vi "data save(1).vi"(8 "error in":errorcluster caption="Error In", 10 "保存时间间隔":u16(ring)=1 items=["无间隔"=1, "1分钟"=60, "5分钟"=300, "10分钟"=600, "30分钟"=1800, "1小时"=3600], 11 "CalData":T1(array[cluster])) -> (0 "error out":errorcluster caption="Error out")   [LabVIEW 2011]
panel:
  in  "targer":enum16{"主舱外回路", "主舱内回路", "实验舱外回路", "实验舱内回路"}(ring)
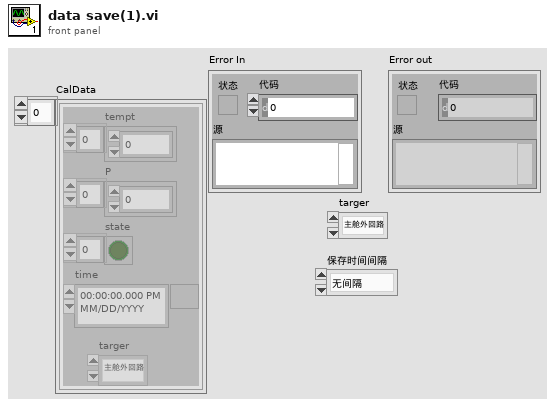
[diagram p1: front panel]
types:
  T1 = cluster{"tempt":dbl[], "P":dbl[], "state":bool[], "time":timestamp, "targer":enum16{"主舱外回路", "主舱内回路", "实验舱外回路", "实验舱内回路"}}[]
  T2 = typedef "Enum File IO - FGV(V)_Ctrls-某型振动实验台测试系统.ctl" = enum16{"New", "Open", "Write Info", "Write Data", "Read Info", "Read Chan Names", "Read Data", "Close", "None"}
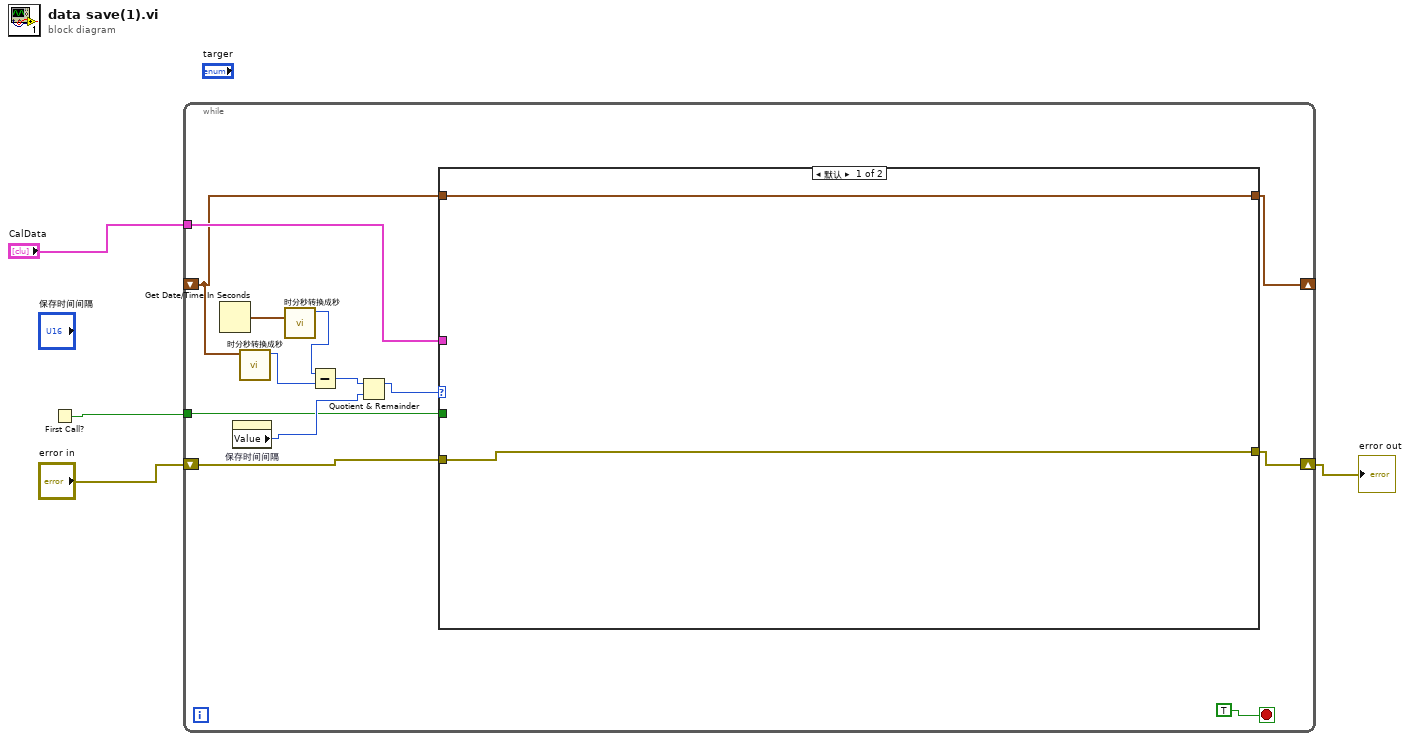
[diagram p0: block diagram]
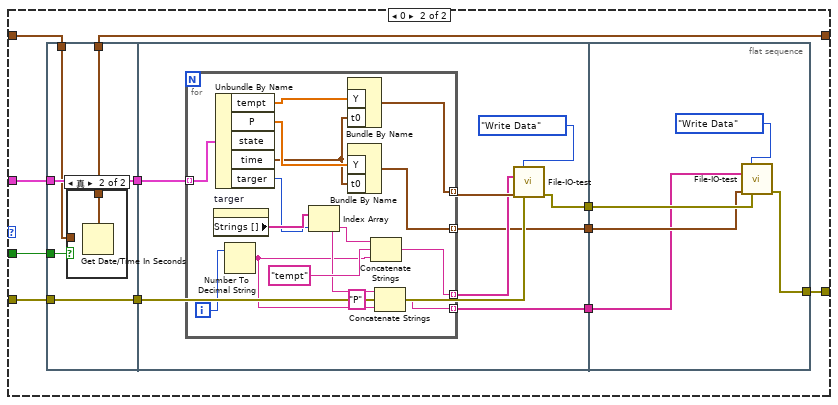
[diagram p2: hidden frame]
diagram:
  n1 = First Call?() -> (First Call?: T/F=w1:bool)
  n2 = while {
    tunnel: "CalData" -> [w17]
    shift-right: [w15] -> w2
    shift-left: "error in" -> [w16]
    shift-right: [w14] -> _
    shift-left: _ -> [w10]
    tunnel: w1 -> [w5]
    stop <- TRUE stop-if-true
    n3 = Get Date/Time In Seconds() -> (seconds since 1Jan1904=w12:timestamp)
    n4 = property on="保存时间间隔" class="Ring (严格)"() -> ("Value"=w7:u16)  [unwired: 2 in, 2 out]
    n5 = call "时分秒转换成秒.vi"("seconds since 1Jan1904"=w10) -> ("数值"=w9:i32)  [unwired: 10 in]
    n6 = call "时分秒转换成秒.vi"("seconds since 1Jan1904"=w12) -> ("数值"=w11:i32)  [unwired: 10 in]
    n7 = Subtract(x=w11, y=w9) -> (x-y=w8:i32)
    n8 = Quotient & Remainder(x=w8, y=w7) -> (x-y*floor(x/y)=w6:i32)  [unwired: 1 out]
    n9 = case shown="默认" w6 {
      tunnel: w17 -> [_ w27]
      tunnel: w16 -> [w19 w26]
      tunnel: [w19 w25] -> w15
      tunnel: [w18 w22] -> w14
      tunnel: w10 -> [w18 w20]
      tunnel: w5 -> [_ w21]
      frame Default {
      }
      frame 0 {
        n10 = flat-sequence {
          tunnel: w26 -> [w34]
          tunnel: w27 -> [w35]
          tunnel: [w35] -> w24
          tunnel: [w34] -> w23
          tunnel: [w32] -> w22
          tunnel: w21 -> [w33]
          tunnel: w20 -> [w31]
          tunnel: [w41] -> w30
          tunnel: [w39] -> w29
          tunnel: [w38] -> w28
          tunnel: w24 -> [w45]
          tunnel: w23 -> [w42]
          tunnel: w30 -> [w64]
          tunnel: [w63] -> w25
          tunnel: w29 -> [w62]
          tunnel: w28 -> [w61]
          frame #0 {
            n11 = case shown="真" w33 {
              tunnel: [w36 w37] -> w32
              tunnel: w31 -> [w36 _]
              frame False {
              }
              frame True {
                n12 = Get Date/Time In Seconds() -> (seconds since 1Jan1904=w37:timestamp)
              }
            }
          }
          frame #1 {
            n13 = for {
              tunnel: w45 -> [w60] mode=indexing
              tunnel: [w57] -> w43 mode=indexing
              tunnel: [w56] -> w39 mode=indexing
              tunnel: [w51] -> w40 mode=indexing
              tunnel: [w47] -> w38 mode=indexing
              i -> [w53]
              n14 = property on="targer" class="Enum (严格)"() -> ("Strings []"=w55:string[])  [unwired: 2 in, 2 out]
              n15 = Unbundle By Name(w60) -> ("tempt"=w59:dbl[], "P"=w58:dbl[], "time"=w46:timestamp, "targer"=w54:enum16{"主舱外回路", "主舱内回路", "实验舱外回路", "实验舱内回路"})  [unwired: 1 out]
              n16 = Number To Decimal String(number=w53) -> (decimal integer string=w49:string)  [unwired: 1 in]
              n17 = Index Array(array=w55, index=w54) -> (element=w50:string)
              n18 = Bundle By Name("Y"=w59, "t0"=w46) -> (w57:waveform(dbl))  [unwired: 1 in]
              n19 = Bundle By Name("Y"=w58, "t0"=w46) -> (w56:waveform(dbl))  [unwired: 1 in]
              n20 = Concatenate Strings(w50, "tempt" ("字符串"), w49) -> (w51:string)
              n21 = Concatenate Strings(w50, "P" ("字符串"), w49) -> (w47:string)
            }
            n22 = call "File-IO-test.vi"("Operation"=Enum_File_IO_-_FGV(V)_Ctrls-某型振动实验台测试系统."Write Data", "Vibration Channel Name Input"=w40, "Vibration Waveform"=w43, "error in"=w42) -> ("error out"=w41:errorcluster)  [unwired: 8 in, 3 out]
          }
          frame #2 {
            n23 = call "File-IO-test.vi"("Operation"=Enum_File_IO_-_FGV(V)_Ctrls-某型振动实验台测试系统."Write Data", "Vibration Channel Name Input"=w61, "Vibration Waveform"=w62, "error in"=w64) -> ("error out"=w63:errorcluster)  [unwired: 8 in, 3 out]
          }
        }
      }
    }
  }
  "error out" <- w2
